vi "Read_generic_GPS_subVI.vi"(10 "Baud Rate":dbl=4800.0, 11 "VISA resource name":refnum<visa-resource-name>="COM6") -> (0 "Longitude W":dbl format="%#_11g", 1 "GPS\nSeconds":dbl=4.0, 2 "GPS\nHour":dbl=3.0, 3 "GPS JD":dbl=150.1250462962963 format="%#_9g", 4 "Latitude N":dbl format="%#_9g", 5 "GPS\nDay":dbl=150.0, 7 "GPS\nMinute":dbl)   [LabVIEW 2021]
doc: "This example application decodes the most common NMEA 0183 Version 3.0 sentence transmitted by GPS receivers, the $GPRMC sentence. The course track is plotted on the screen, while the ground speed and course heading are also displayed.\n\nThe \"Read NMEA GPS SubVI.vi\" returns time, position, ground speed, and magnetic variation. This subVI initializes the serial port on first call. On subsequent calls, the initialization is skipped. Always use the Stop input when stopping the subVI so that the serial port connection is closed. This subVI is suitable for use in LabVIEW Real-Time applications (normal priority loop), and uses the VISA serial API. \n\nIn your GPS interface configuration, use the \"NMEA OUT\" setting and set the baud rate to the default 4800 bps setting. Connect your GPS unit to the computer or LabVIEW Real-Time target serial port using a PC Interface Cable, available from the GPS vendor. \n\nThis example should work with any NMEA 0183 compatible GPS unit. The example was developed and tested using a Garmin eTrex GPS unit."
uses:
  Compass.ctl
  Instance           4 24Saved   Read_generic_GPS .vi
panel:
  out "Speed over ground  (knots)":dbl(knob) scale=0.0..28.0
  out "Course over ground (degrees)":T1=47 scale=0.0..360.0
  out "XY Graph":cluster{"Y":dbl[], "Y":dbl[]}[](graph)
  out "error out":errorcluster
  out "GPS Data":T2={"UTC Time"=timestamp(3263338804 s since 1904-01-01), "Local Time"=timestamp(3263320804 s since 1904-01-01), "Lattitude (ddmm.mmmm)"=4839.21326, "Lattitude North/South"="N", "Longitude (ddmm.mmmm)"=12327.15147, "Longitude East/West"="W", "Magnetic Variation (degrees)"=0.0, "Variation East/West"="", "Speed over ground (knots)"=0.0, "Course over ground (degrees)"=46.63} {"Course over ground (degrees)" format="%#.6g"; "Speed over ground (knots)" format="%#.6g"; "Magnetic Variation (degrees)" format="%#.6g"; "Longitude (ddmm.mmmm)" format="%#.6g"; "Lattitude (ddmm.mmmm)" format="%#.6g"}
  out "GPS Data Valid?":bool=TRUE
  in  "stop":bool
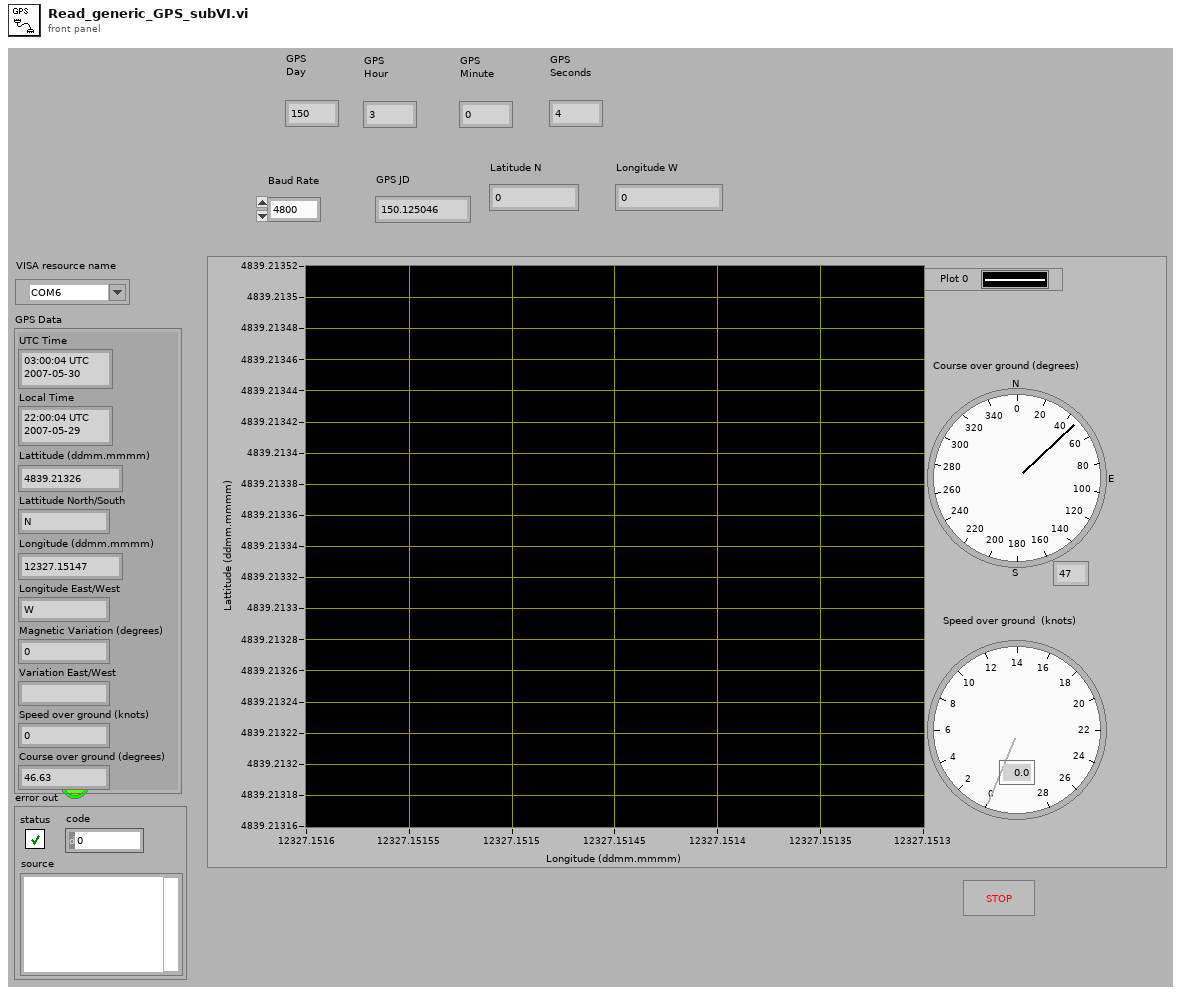
[diagram p1: front panel]
types:
  T1 = typedef "Compass.ctl" = i32
  T2 = cluster{"UTC Time":timestamp, "Local Time":timestamp, "Lattitude (ddmm.mmmm)":dbl, "Lattitude North/South":string, "Longitude (ddmm.mmmm)":dbl, "Longitude East/West":string, "Magnetic Variation (degrees)":dbl, "Variation East/West":string, "Speed over ground (knots)":dbl, "Course over ground (degrees)":dbl}
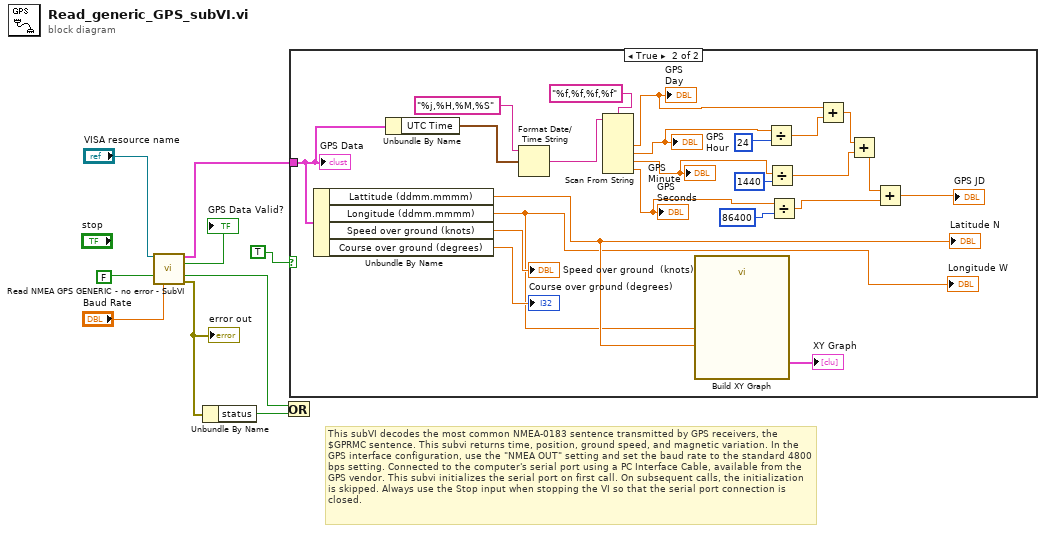
[diagram p0: block diagram]
diagram:
  # "This subVI decodes the most common NMEA-0183 sentence transmitted by GPS receivers, the $GPRMC sentence. This subvi returns time, position, ground speed, and magnetic variation. In the GPS interface configuration, use the \"NMEA OUT\" setting and set the baud rate to the standard 4800 bps setting. Connected to the computer's serial port using a PC Interface Cable, available from the GPS vendor. This subvi initializes the serial port on first call. On subsequent calls, the initialization is skipped. Always use the Stop input when stopping the VI so that the serial port connection is closed."
  n1 = call "Read NMEA GPS GENERIC - no error - SubVI.vi"("VISA resource name"="VISA resource name", "stop"=FALSE, "Baud Rate"="Baud Rate") -> ("GPS $GPRMC Data"=w8:T2, "GPS Data Valid?"=→"GPS Data Valid?":bool, "Stopped?"=w5:bool, "error out"=w7:errorcluster)  [unwired: 9 in]
  "error out" <- w7
  n2 = Unbundle By Name(w7) -> ("status"=w6:bool)
  n3 = Or(x=w5, y=w6) -> ()  [unwired: 1 out]
  n4 = case shown="True" TRUE {
    tunnel: w8 -> [_ w29]
    frame False {
    }
    frame True {
      n5 = Unbundle By Name(w29) -> ("Lattitude (ddmm.mmmm)"=w12:dbl, "Longitude (ddmm.mmmm)"=w11:dbl, "Speed over ground (knots)"=→"Speed over ground  (knots)":dbl, "Course over ground (degrees)"=→"Course over ground (degrees)":dbl)
      "Latitude N" <- w12
      "Longitude W" <- w11
      n6 = Unbundle By Name(w29) -> ("UTC Time"=w28:timestamp)
      n7 = Format Date/Time String(time format string (%c)="%j,%H,%M,%S", seconds (now)=w28) -> (date/time string=w26:string)  [unwired: 1 in]
      n8 = Scan From String(format string="%f,%f,%f,%f", input string=w26) -> (output 1=w18:dbl, output 2=w19:dbl, output 3=w20:dbl, output 4=w21:dbl)  [unwired: 6 in, 3 out]
      "GPS\nDay" <- w18
      "GPS\nHour" <- w19
      "GPS\nMinute" <- w20
      "GPS\nSeconds" <- w21
      n9 = call "Build XY Graph"("Y Input"=w12, "X Input"=w11) -> ("XY Graph"=→"XY Graph":cluster{"Y":dbl[], "Y":dbl[]}[])  [unwired: 8 in, 1 out]
      n10 = Divide(x=w19, y=24) -> (x/y=w17:dbl)
      n11 = Divide(x=w20, y=1440) -> (x/y=w15:dbl)
      n12 = Divide(x=w21, y=86400) -> (x/y=w13:dbl)
      n13 = Add(x=w18, y=w17) -> (x+y=w16:dbl)
      n14 = Add(x=w16, y=w15) -> (x+y=w14:dbl)
      n15 = Add(x=w14, y=w13) -> (x+y=→"GPS JD":dbl)
      "GPS Data" <- w29
    }
  }
